vi "ExSubPickStrip.vi"(2 "error in (no error)":errorcluster, 3 "Strip to display":u32, 4 "Camera Handle":u32) -> (0 "error out":errorcluster, 1 "Camera Handle":u32)   [LabVIEW 2010]
panel:
  # "ExSubPickStrip:\nThis sub-VI is given a strip number\nthen programs the camera to return\nthis strip only (strip and row are same)."
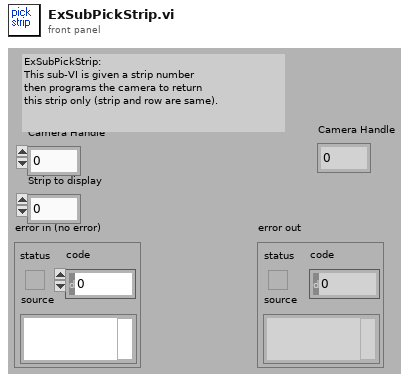
[diagram p1: front panel]
types:
  T1 = cluster{"X begin, start at beginning of strip":i32, "Xdim":u32, "Bin by 1 in both X and Y ":i32, "Strip to display":u32, "Strip to display":u32, "Bin by 1 in both X and Y ":i32}
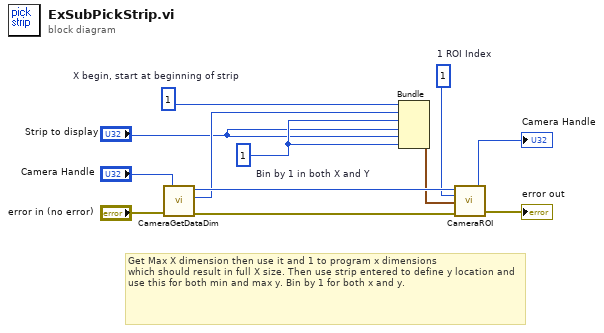
[diagram p0: block diagram]
diagram:
  w5 = 1  # 1 ROI Index
  w7 = 1  # Bin by 1 in both X and Y
  w2 = 1  # X begin, start at beginning of strip
  # "Get Max X dimension then use it and 1 to program x dimensions\nwhich should result in full X size. Then use strip entered to define y location and use this for both min and max y. Bin by 1 for both x and y."
  n1 = call <userlib>:"CameraGetDataDim.vi"("Camera Handle"="Camera Handle", "error in"="error in (no error)") -> ("Camera Handle"=w11:u32, "Xdim"=w8:u32, "error out"=w9:errorcluster)  [unwired: 1 out]
  n2 = Bundle("X begin, start at beginning of strip"=w2, "Xdim"=w8, "Bin by 1 in both X and Y"=w7, "Strip to display"="Strip to display", "Strip to display"="Strip to display", "Bin by 1 in both X and Y"=w7) -> (w6:T1)  [unwired: 1 in]
  n3 = call <userlib>:"CameraROI.vi"("error in"=w9, "ROI Params"=w6, "ROI Index"=w5, "Camera Handle"=w11) -> ("error out"=→"error out":errorcluster, "Camera Handle"=→"Camera Handle":u32)
